vi "Write Home.vi"(8 "error in (no error)":errorcluster, 10 "Home":i8, 11 "Amphipod in":refnum<class "Amphipod.lvclass">) -> (0 "error out":errorcluster, 3 "Amphipod out":refnum<class "Amphipod.lvclass">)   [LabVIEW 2019, in "23.lvlib" / "Amphipod.lvclass"]
uses:
  Amphipod.lvclass
  Amphipod.lvclass/Amphipod.ctl
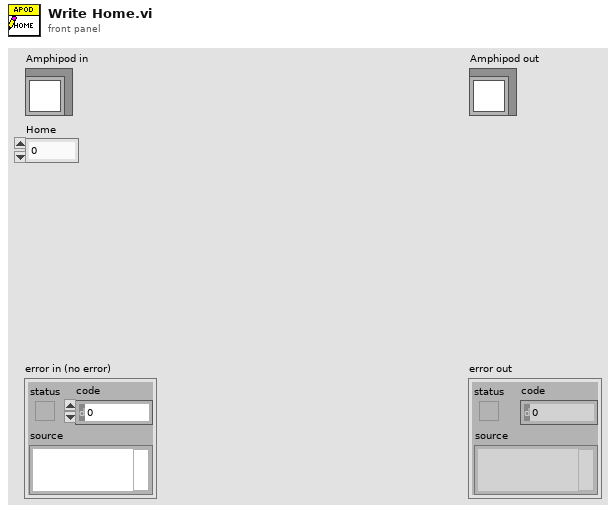
[diagram p1: front panel]
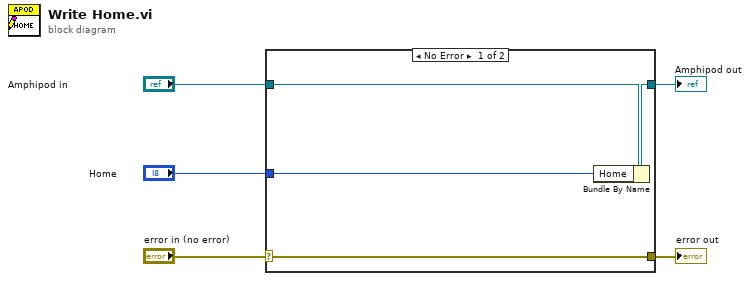
[diagram p0: block diagram]
diagram:
  n1 = case shown="No Error" "error in (no error)" {
    selector: "error in (no error)" -> [w9 w10]
    tunnel: [w9 w10] -> w4
    tunnel: [w7 w11] -> w2
    tunnel: "Amphipod in" -> [w8 w11]
    tunnel: "Home" -> [w6 _]
    frame No Error {
      n2 = Bundle By Name(cluster=w8, "Home"=w6) -> (w7:refnum<class "Amphipod.lvclass">)
    }
    frame Error {
    }
  }
  "error out" <- w4
  "Amphipod out" <- w2
